vi "set_ref_clus_MagPS.vi"(6 "input cluster":T1, 9 "level_LN2":dbl, 10 "level_LHe":dbl, 11 "status":bool) -> ()   [LabVIEW 2019]
uses:
  cluster_ref_MagPS.ctl
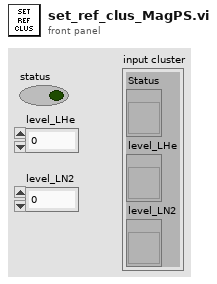
[diagram p1: front panel]
types:
  T1 = typedef "cluster_ref_MagPS.ctl" = cluster{"Status":refnum<vi>, "level_LHe":refnum<vi>, "level_LN2":refnum<vi>}
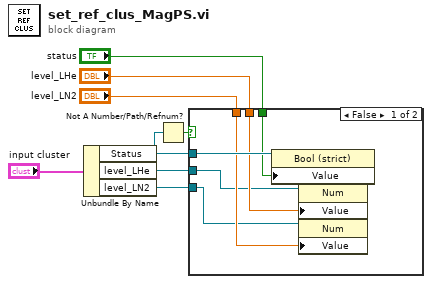
[diagram p0: block diagram]
diagram:
  n1 = Unbundle By Name("input cluster") -> ("Status"=w7:refnum<vi>, "level_LHe"=w6:refnum<vi>, "level_LN2"=w5:refnum<vi>)
  n2 = Not A Number/Path/Refnum?(number/path/refnum=w7) -> (NaN/Path/Refnum?=w8:bool)
  n3 = case shown="False" w8 {
    tunnel: w7 -> [w14 _]
    tunnel: w6 -> [w9 _]
    tunnel: w5 -> [w11 _]
    tunnel: "status" -> [w13 _]
    tunnel: "level_LHe" -> [w10 _]
    tunnel: "level_LN2" -> [w12 _]
    frame False {
      n4 = property class="Bool (strict)"(reference=w14, "Value"=w13) -> ()  [unwired: 1 in, 2 out]
      n5 = property class="Num"(reference=w9, "Value"=w10) -> ()  [unwired: 1 in, 2 out]
      n6 = property class="Num"(reference=w11, "Value"=w12) -> ()  [unwired: 1 in, 2 out]
    }
    frame True {
    }
  }
